vi "Plot Initialize.vi"(5 "Plot Legend Color":u32(colorbox), 6 "Control Ref Cluster":T1, 7 "Main Frame Color":u32(colorbox), 8 "error in (no error)":errorcluster, 11 "2D Compass.lvclass in":refnum<class "2D Compass.lvclass">) -> (0 "error out":errorcluster, 3 "2D Compass.lvclass out":refnum<class "2D Compass.lvclass">)   [LabVIEW 2017, in "2D Compass.lvclass"]
uses:
  <vilib>/Math Plots/2D Math Plots/2D Compass/2D Compass/2D Compass.lvclass
  <vilib>/Math Plots/2D Math Plots/2D Plot/Action String/2DMathPlot Ctrl Act Cluster.ctl
  <vilib>/Math Plots/2D Math Plots/2D Plot/Action String/2DMathPlot State Class.ctl
  <vilib>/Math Plots/2D Math Plots/2D Plot/2D Plot/2D Plot.lvclass
  <vilib>/Math Plots/Plot Private Lib/NI_Math Plot Private Lib.lvlib
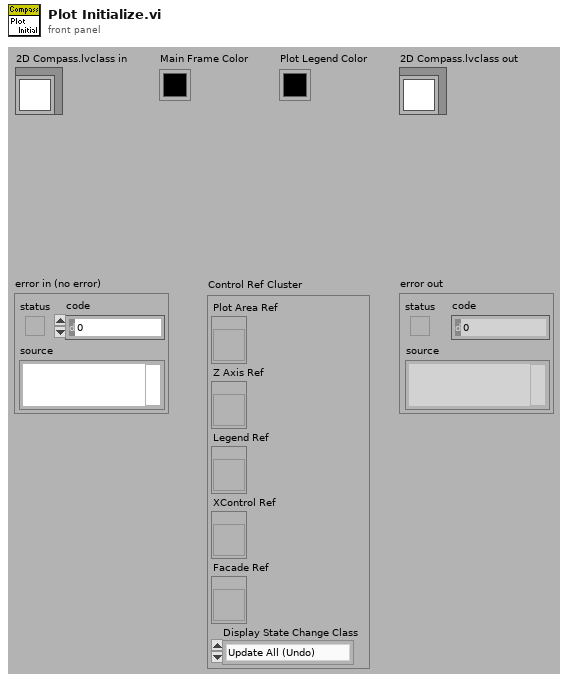
[diagram p1: front panel]
types:
  T1 = typedef "2DMathPlot Ctrl Act Cluster.ctl" = cluster{"Plot Area Ref":refnum<vi>, "Z Axis Ref":refnum<vi>, "Legend Ref":refnum<vi>, "XControl Ref":refnum<vi>, "Facade Ref":refnum<vi>, "Display State Change Class":T2}
  T2 = typedef "2DMathPlot State Class.ctl" = enum16{"Update All (Undo)", "Update General", "Update Appearance", "Update Format", "Update Scale", "Update Marker", "Update Cursor", "None"}
  T3 = typedef "LVRectTypeDef.ctl" = cluster{"Left":i16, "Top":i16, "Right":i16, "Bottom":i16}
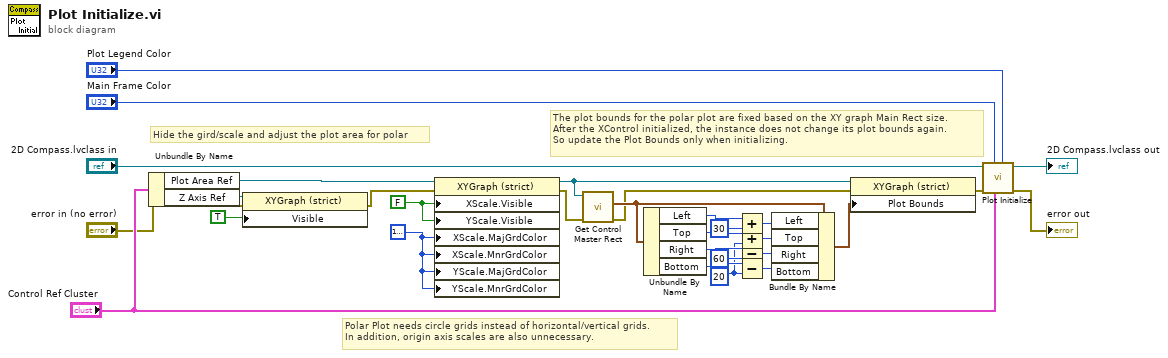
[diagram p0: block diagram]
diagram:
  w13 = i16 20 ("y")
  w24 = u32 16777216 ("X Scale.Grid Colors:Major Color")
  w25 = FALSE ("X Scale.Visible")
  # "The plot bounds for the polar plot are fixed based on the XY graph Main Rect size.\nAfter the XControl initialized, the instance does not change its plot bounds again.\nSo update the Plot Bounds only when initializing."
  # "Polar Plot needs circle grids instead of horizontal/vertical grids.\nIn addition, origin axis scales are also unnecessary."
  # "Hide the gird/scale and adjust the plot area for polar"
  n1 = Unbundle By Name("Control Ref Cluster") -> ("Plot Area Ref"=w29:refnum<vi>, "Z Axis Ref"=w9:refnum<vi>)
  n2 = property class="XYGraph (strict)"(reference=w9, error in="error in (no error)", "Visible"=TRUE) -> (error out=w7:errorcluster)  [unwired: 1 out]
  n3 = property class="XYGraph (strict)"(reference=w29, error in=w7, "XScale.Visible"=w25, "YScale.Visible"=w25, "XScale.MajGrdColor"=w24, "XScale.MnrGrdColor"=w24, "YScale.MajGrdColor"=w24, "YScale.MnrGrdColor"=w24) -> (reference out=w6:refnum<vi>, error out=w4:errorcluster)
  n4 = call <vilib>:"Get Control Master Rect.vi"("error in (no error)"=w4, "reference"=w6) -> ("error out"=w3:errorcluster, "Master Bounds Rect"=w5:T3)  [unwired: 8 out]
  n5 = Unbundle By Name(w5) -> ("Left"=w22:i16, "Top"=w19:i16, "Right"=w17:i16, "Bottom"=w16:i16)
  n6 = Add(x=w22, y=i16 30) -> (x+y=w20:i16)
  n7 = Add(x=w19, y=w13) -> (x+y=w18:i16)
  n8 = Subtract(x=w17, y=i16 60) -> (x-y=w12:i16)
  n9 = Subtract(x=w16, y=w13) -> (x-y=w15:i16)
  n10 = Bundle By Name(cluster=w5, "Left"=w20, "Top"=w18, "Right"=w12, "Bottom"=w15) -> (w23:T3)
  n11 = property class="XYGraph (strict)"(reference=w6, error in=w3, "Plot Bounds"=w23) -> (error out=w11:errorcluster)  [unwired: 1 out]
  n12 = call-parent "Plot Initialize.vi"("Plot Legend Color"="Plot Legend Color", "Control Ref Cluster"="Control Ref Cluster", "Main Frame Color"="Main Frame Color", "error in (no error)"=w11, "2D Plot.lvclass in"="2D Compass.lvclass in") -> ("error out"=→"error out":errorcluster, "2D Plot.lvclass out"=→"2D Compass.lvclass out":refnum<class "2D Compass.lvclass">)  [unwired: 5 out]
